vi "Setpoint.vi"(8 "error in (no error)":errorcluster, 10 "Setpoint [A]":dbl format="%.5f", 11 "PS Driver.lvlib:PS Driver.lvclass in":refnum<class "PS Driver.lvclass">) -> (0 "error out":errorcluster, 2 "Setpoint out (A)":dbl, 3 "PS Driver.lvlib:PS Driver.lvclass out":refnum<class "PS Driver.lvclass">)   [LabVIEW 2019, in "PS Driver.lvlib" / "PS Driver.lvclass"]
uses:
  PS Driver.lvclass
  PS Driver.lvclass/PS Driver.ctl
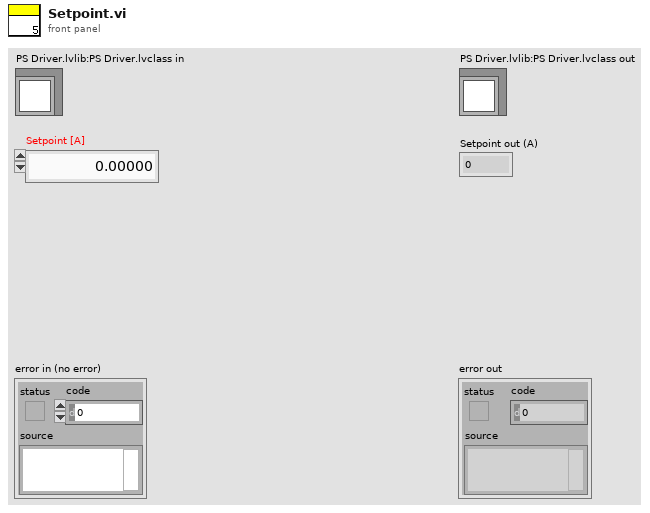
[diagram p1: front panel]
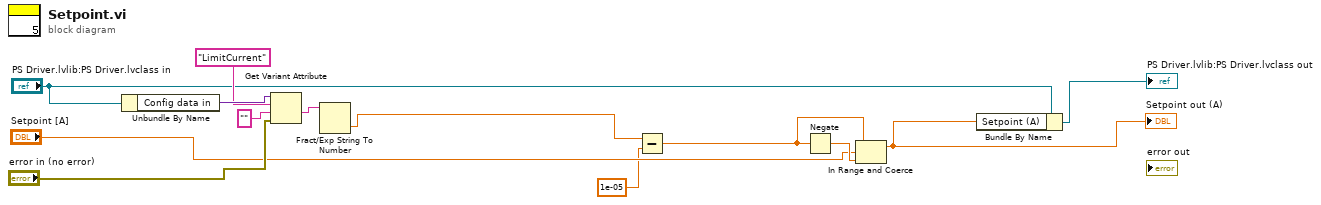
[diagram p0: block diagram]
diagram:
  n1 = Unbundle By Name("PS Driver.lvlib:PS Driver.lvclass in") -> ("Config data in"=w13:variant)
  n2 = Get Variant Attribute(Variant=w13, name="LimitCurrent", default value (empty Variant)="", error in="error in (no error)") -> (value=w9:string)  [unwired: 3 out]
  n3 = Fract/Exp String To Number(string=w9) -> (number=w1:dbl)  [unwired: 3 in, 1 out]
  n4 = Subtract(x=w1, y=1e-05) -> (x-y=w5:dbl)
  n5 = Negate(x=w5) -> (-x=w8:dbl)
  n6 = In Range and Coerce(upper limit=w5, x="Setpoint [A]", lower limit=w8) -> (coerced(x)=w2:dbl)  [unwired: 1 out]
  "Setpoint out (A)" <- w2
  n7 = Bundle By Name(cluster="PS Driver.lvlib:PS Driver.lvclass in", "Setpoint (A)"=w2) -> (→"PS Driver.lvlib:PS Driver.lvclass out":refnum<class "PS Driver.lvclass">)
